vi "Rotate_vector_numeric.vi"(9 "Angle (deg)":sgl, 10 "Numeric 4":sgl, 11 "Numeric 3":sgl) -> (2 "Numeric":dbl, 3 "Numeric 2":dbl)   [LabVIEW 2014]
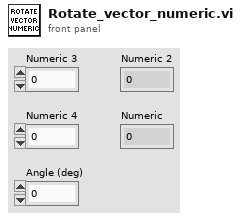
[diagram p1: front panel]
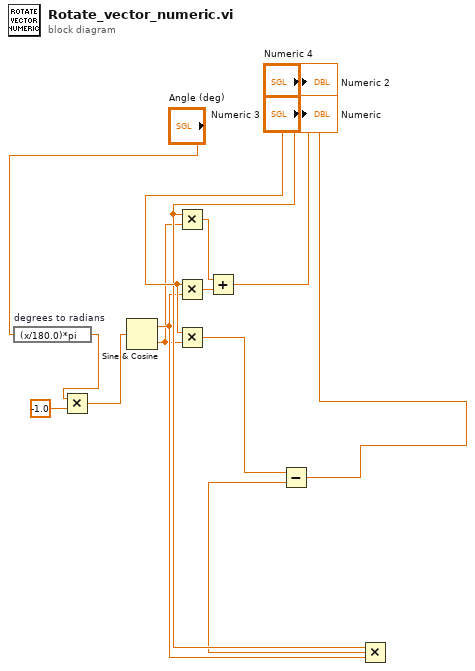
[diagram p0: block diagram]
diagram:
  n1 = expression code="(x/180.0)*pi" "degrees to radians"("Angle (deg)") -> (w13:sgl)
  n2 = Multiply(x=w13, y=-1.0) -> (x*y=w14:dbl)
  n3 = Sine & Cosine(0:w14) -> (1:w2:dbl, 2:w1:dbl)
  n4 = Multiply(x="Numeric 4", y=w1) -> (x*y=w3:dbl)
  n5 = Multiply(x="Numeric 3", y=w2) -> (x*y=w4:dbl)
  n6 = Multiply(x="Numeric 3", y=w1) -> (x*y=w5:dbl)
  n7 = Add(x=w3, y=w4) -> (x+y=→"Numeric 2":dbl)
  n8 = Multiply(x="Numeric 4", y=w2) -> (x*y=w6:dbl)
  n9 = Subtract(x=w5, y=w6) -> (x-y=→"Numeric":dbl)
